vi "Query Model.vi"(8 "error in (no error)":errorcluster, 11 "VISA resource name":refnum<visa-resource-name>) -> (0 "error out":errorcluster, 2 "Model":i32(ring) items=["", "DMM6500", "DAQ6510"], 3 "VISA resource name out":refnum<visa-resource-name>)   [LabVIEW 2023, in "Keithley DMM6500 DAQ6500 Series.lvlib"]
doc: "Queries instrument and returns model in use."
uses:
  <instrlib>/Keithley DMM6500 DAQ6500 Series/Keithley DMM6500 DAQ6500 Series.lvlib
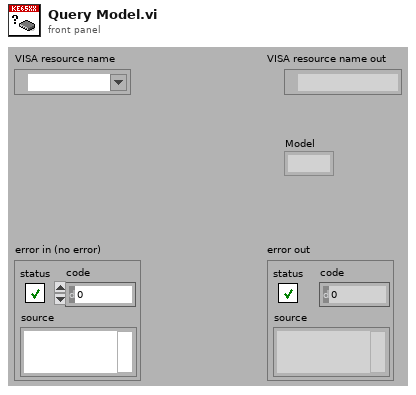
[diagram p1: front panel]
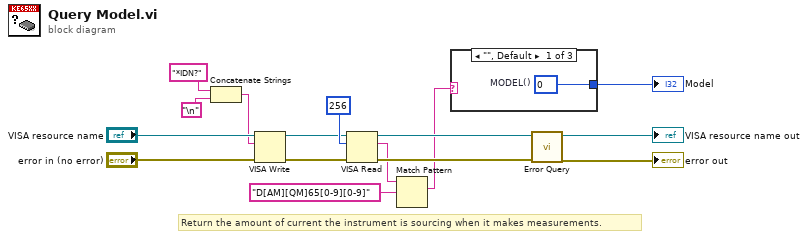
[diagram p0: block diagram]
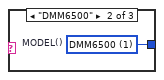
[diagram p2: hidden frame]
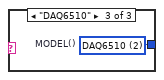
[diagram p3: hidden frame]
diagram:
  # "Return the amount of current the instrument is sourcing when it makes measurements."
  n1 = Concatenate Strings("*IDN?" ("string"), "\n") -> (w4:string)
  n2 = VISA Write(VISA resource name="VISA resource name", write buffer=w4, error in (no error)="error in (no error)") -> (VISA resource name out=w10:refnum<visa-resource-name>, error out=w13:errorcluster)  [unwired: 1 out]
  n3 = VISA Read(VISA resource name=w10, byte count=u32 256, error in (no error)=w13) -> (VISA resource name out=w9:refnum<visa-resource-name>, read buffer=w3:string, error out=w12:errorcluster)  [unwired: 1 out]
  n4 = Match Pattern(string=w3, regular expression="D[AM][QM]65[0-9][0-9]") -> (match substring=w2:string)  [unwired: 1 in, 3 out]
  n5 = case shown="\"\", Default" w2 {
    tunnel: [w17 w18 w19] -> w1
    frame "", Default {
      w17 = 0 items=["", "DMM6500", "DAQ6510"]  # MODEL()
    }
    frame "DMM6500" {
      w18 = 1 items=["", "DMM6500", "DAQ6510"]  # MODEL()
    }
    frame "DAQ6510" {
      w19 = 2 items=["", "DMM6500", "DAQ6510"]  # MODEL()
    }
  }
  "Model" <- w1
  n6 = call <instrlib>:"Error Query.vi"("error in (no error)"=w12, "VISA resource name"=w9) -> ("error out"=→"error out":errorcluster, "VISA resource name out"=→"VISA resource name out":refnum<visa-resource-name>)  [unwired: 6 in, 2 out]
